vi "SerialSettings.vi"(7 "Operation":T2, 8 "error in (no error)":errorcluster, 11 "Serial Info":T1={"Port"="", "baud rate"=9600, "data bits"=8, "stop bits"=10, "parity"=enum."None", "flow control"=0} {"flow control" items=["None", "XON/XOFF", "RTS/CTS", "XON/XOFF & RTS/CTS", "DTR/DSR", "XON/XOFF & DTR/DSR"]; "stop bits" items=["1.0"=10, "1.5"=15, "2.0"=20]; "data bits" min=5 max=8 step=1}) -> (0 "error out":errorcluster, 3 "Serial Info Out":T1={"Port"="", "baud rate"=9600, "data bits"=8, "stop bits"=10, "parity"=enum."None", "flow control"=0} {"flow control" items=["None", "XON/XOFF", "RTS/CTS", "XON/XOFF & RTS/CTS", "DTR/DSR", "XON/XOFF & DTR/DSR"]; "stop bits" items=["1.0"=10, "1.5"=15, "2.0"=20]; "data bits" min=5 max=8 step=1})   [LabVIEW 2011]
uses:
  Strict Type Controls/Settings Operation.ctl
  <vilib>/Utility/config.llb/NI_LVConfig.lvlib
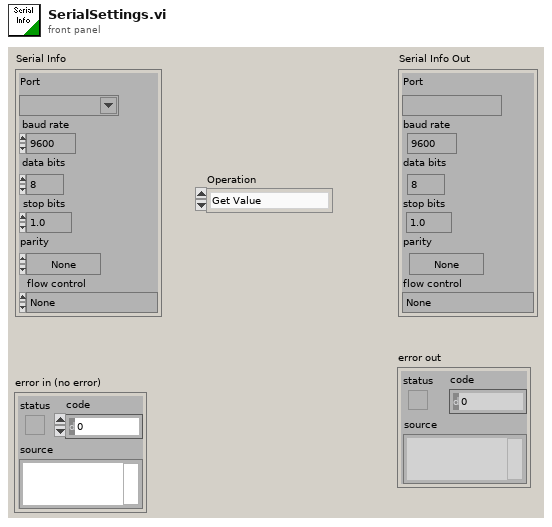
[diagram p1: front panel]
types:
  T1 = cluster{"Port":refnum<visa-resource-name>, "baud rate":u32, "data bits":u16, "stop bits":u16, "parity":enum16{"None", "Odd", "Even", "Mark", "Space"}, "flow control":u16}
  T2 = typedef "Settings Operation.ctl" = enum8{"Get Value", "Set Value", "Read File", "Write File", "Write Stored Value"}
  T3 = typedef "NI_LVConfig.lvlib/Config Data RefNum.ctl" = refnum<k1>
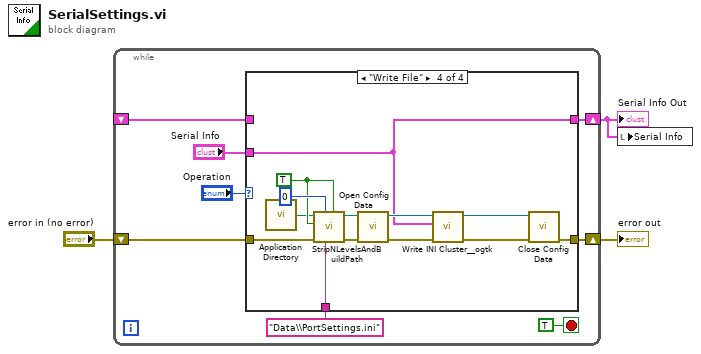
[diagram p0: block diagram]
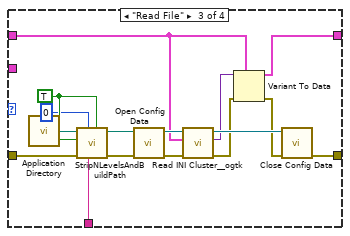
[diagram p4: hidden frame]
diagram:
  n1 = while {
    shift-right: [w10] -> w1
    shift-left: _ -> [w11]
    shift-right: [w8] -> w2
    shift-left: "error in (no error)" -> [w9]
    stop <- TRUE stop-if-true
    n2 = case shown="\"Write File\"" "Operation" {
      tunnel: w11 -> [w13 _ w19 _]
      tunnel: [w13 w15 w18 w32] -> w10
      tunnel: "Serial Info" -> [_ w15 _ w32]
      tunnel: w9 -> [w12 w14 w30 w43]
      tunnel: [w12 w14 w31 w44] -> w8
      tunnel: "Data\\PortSettings.ini" ("Build Path") -> [_ _ w27 w42]
      frame "Get Value", Default {
      }
      frame "Set Value" {
      }
      frame "Read File" {
        w25 = TRUE ("Is File?")
        n3 = call <vilib>:"Application Directory.vi"() -> ("Application Directory"=w26:path)
        n4 = call "StripNLevelsAndBuildPath.vi"("Create Folders"=w25, "Build Path"=w27, "Strip Levels"=0, "error in(no error)"=w30, "Is File"=w25, "Path In"=w26) -> ("error out"=w29:errorcluster, "Path Out"=w28:path)  [unwired: 4 in]
        n5 = call <vilib>:"Open Config Data.vi"("error in (no error)"=w29, "configuration file path"=w28) -> ("error out"=w22:errorcluster, "refnum"=w23:T3)  [unwired: 7 in, 1 out]
        n6 = call <userlib>:"Read INI Cluster__ogtk.vi"("error in (no error)"=w22, "INI Fomatted Cluster Type"=w19, "refnum"=w23) -> ("error out"=w17:errorcluster, "INI Fomatted Cluster"=w20:variant, "dup refnum"=w21:T3)  [unwired: 4 in, 2 out]
        n7 = Variant To Data(error in=w17, type=w19, Variant=w20) -> (data=w18:T1, error out=w16:errorcluster)
        n8 = call <vilib>:"Close Config Data.vi"("error in (no error)"=w16, "refnum"=w21) -> ("error out"=w31:errorcluster)  [unwired: 1 in, 8 out]
      }
      frame "Write File" {
        w40 = TRUE ("Is File?")
        n9 = call <vilib>:"Application Directory.vi"() -> ("Application Directory"=w39:path)
        n10 = call "StripNLevelsAndBuildPath.vi"("Create Folders"=w40, "Build Path"=w42, "Strip Levels"=0, "error in(no error)"=w43, "Is File"=w40, "Path In"=w39) -> ("error out"=w38:errorcluster, "Path Out"=w37:path)  [unwired: 4 out]
        n11 = call <vilib>:"Open Config Data.vi"("error in (no error)"=w38, "configuration file path"=w37) -> ("error out"=w35:errorcluster, "refnum"=w36:T3)  [unwired: 7 in, 1 out]
        n12 = call <userlib>:"Write INI Cluster__ogtk.vi"("error in (no error)"=w35, "INI Fomatted Cluster"=w32, "refnum"=w36) -> ("error out"=w33:errorcluster, "dup refnum"=w34:T3)  [unwired: 7 in]
        n13 = call <vilib>:"Close Config Data.vi"("error in (no error)"=w33, "refnum"=w34) -> ("error out"=w44:errorcluster)  [unwired: 1 in, 8 out]
      }
    }
  }
  "error out" <- w2
  "Serial Info Out" <- w1
  n14 = local write "Serial Info"(w1) -> ()
